vi "Calibrate_Test_Sums.vi"(8 "error in (no error)":errorcluster, 11 "StageSelection":enum16{"X-Y", "Z"}(ring)) -> (0 "error out":errorcluster)   [LabVIEW 2020]
doc: "Use this template to create a dialog box with event handling."
uses:
  Globals/gl_Calibration globals.vi
  Typedefs/Top level VI states.ctl
panel:
  out "Znorm_to_um_scaling":dbl
  in  "Delay":u32=1000
  out "Cal":sgl[][](array[numeric])
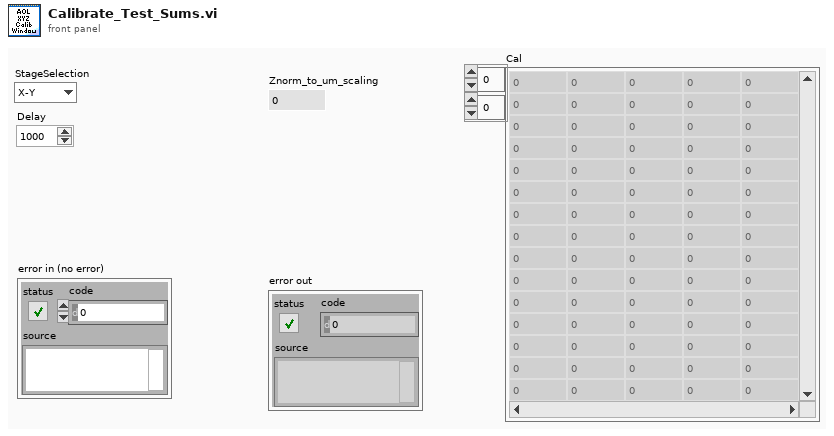
[diagram p1: front panel]
types:
  T1 = typedef "Cal points.ctl" = enum16{"5-points calibration (crude)", "11-points calibration", "21-points calibration", "41-points calibration"}
  T2 = typedef "Top level VI states.ctl" = enum16{"None", "Initialise UI", "<STACK PROTOCOL STATES>", "AOL Zstack-START", "AOL Zstack-STOP", "Motor Zstack-START", "Motor Zstack-STOP", "<ACQUISITION PROTOCOL STATES> ", "Functional Acquisition-START", "Functional Acquisition-STOP", "Single Plane Acquisition-START", "Single Plane Acquisition-STOP", "Volume Acquisition-START", "Volume Acquisition-STOP", "<LIVE IMAGING PROTOCOL STATES>", "Live Imaging-START", "Live Imaging-STOP", "Live Plane Imaging-START", "Live Plane Imaging-STOP", "Live Volume Imaging-START", "Live Volume Imaging-STOP", "<MOVEMENT CORRECTION PROTOCOL STATES>", "EXIT"}
  T3 = typedef "General Scan Parameters.ctl" = cluster{"Field of View":sgl, "Frame Size":u16, "Dwell Time (ms)":dbl, "Wavelength (nm)":dbl, "Zoom":dbl, "AOL Xc":sgl, "AOL Yc":sgl, "AOL Zc":sgl, "AOL Mode":enum16{"Raster", "Structural", "Pointing", "Mini Scan", "Alignment"}, "Imaging Mode":enum16{"Live Imaging", "AOL Zstack", "Motor Zstack", "Functional Imaging"}}
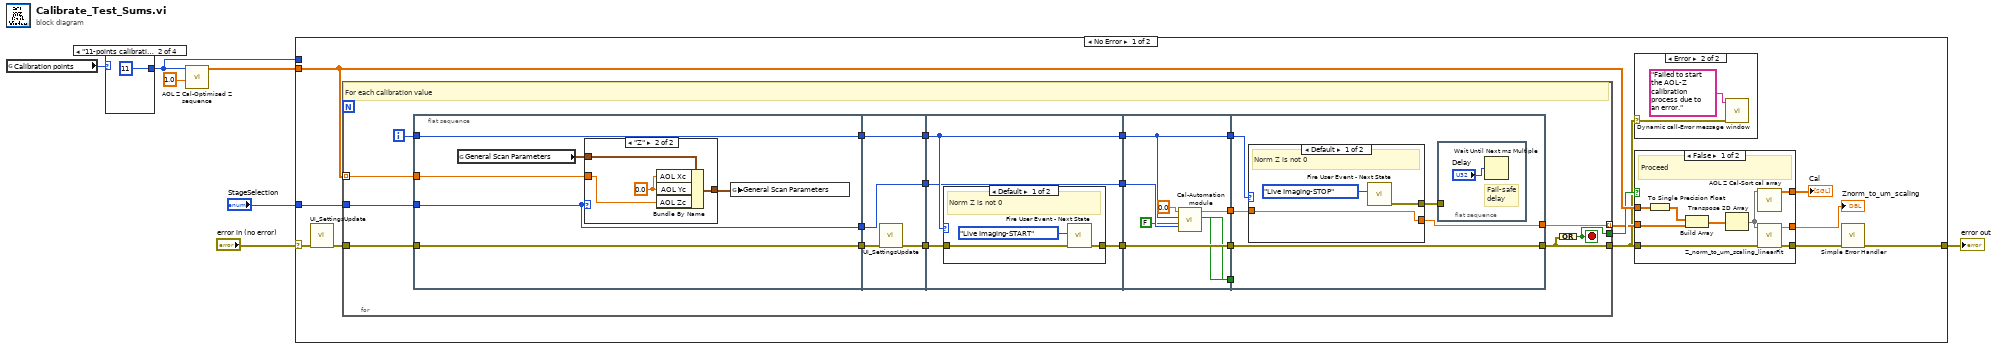
[diagram p0: block diagram]
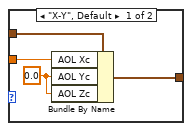
[diagram p2: hidden frame]
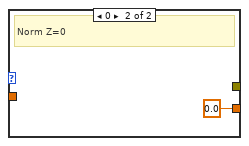
[diagram p4: hidden frame]
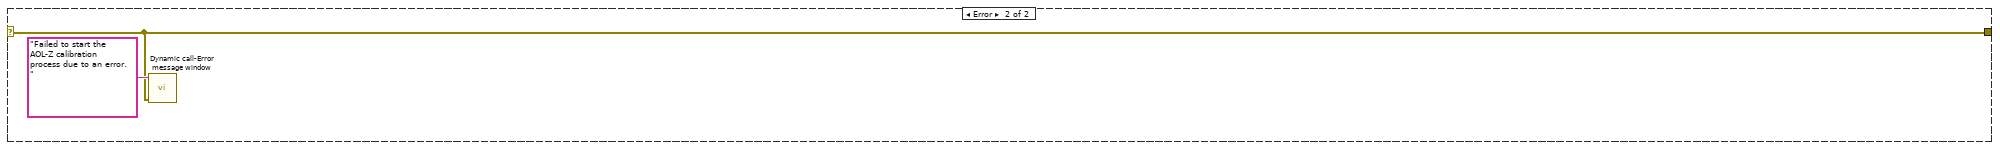
[diagram p7: hidden frame]
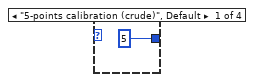
[diagram p8: hidden frame]
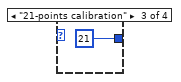
[diagram p9: hidden frame]
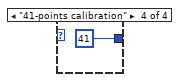
[diagram p10: hidden frame]
diagram:
  n1 = global read "gl_Calibration globals.vi" "Calibration points"() -> (w5:T1)
  n2 = case shown="\"11-points calibration\"" w5 {
    tunnel: [5 ("Calibration points") 11 ("Calibration points") 21 ("Calibration points") 41 ("Calibration points")] -> w4
    frame "5-points calibration (crude)", Default {
    }
    frame "11-points calibration" {
    }
    frame "21-points calibration" {
    }
    frame "41-points calibration" {
    }
  }
  n3 = call "AOL Z Cal-Optimised Z sequence.vi"("Max positive value"=1.0, "Calibration points"=w4) -> ("Calibration's optimised norm Z sequence"=w7:dbl[])  [unwired: 8 in, 1 out]
  n4 = case shown="No Error" "error in (no error)" {
    selector: "error in (no error)" -> [w15 w100]
    tunnel: w7 -> [w22 _]
    tunnel: w4 -> [_ _]
    tunnel: [w18 w100] -> w3
    tunnel: "StageSelection" -> [w13 _]
    frame No Error {
      n5 = call "UI_SettingsUpdate.vi"("error in (no error)"=w15) -> ("error out"=w17:errorcluster)  [unwired: 10 in]
      n6 = for {
        tunnel: w22 -> [w38] mode=indexing
        tunnel: [w43] -> w16 mode=indexing
        tunnel: [w25] -> w19
        tunnel: [w26] -> w14
        tunnel: w17 -> [w34]
        tunnel: w13 -> [w32]
        i -> [w35]
        stop <- w25 stop-if-true
        # "For each calibration value"
        n7 = flat-sequence {
          tunnel: w35 -> [w49]
          tunnel: [w49] -> w39
          tunnel: w38 -> [w45]
          tunnel: w34 -> [w48]
          tunnel: [w48] -> w33
          tunnel: w32 -> [w44]
          tunnel: [w44] -> w28
          tunnel: [w61] -> w41
          tunnel: w39 -> [w61]
          tunnel: w33 -> [w60]
          tunnel: [w59] -> w31
          tunnel: [w58] -> w29
          tunnel: w28 -> [w58]
          tunnel: [w65] -> w42
          tunnel: w41 -> [w65]
          tunnel: [w64] -> w36
          tunnel: w31 -> [w63]
          tunnel: [w62] -> w30
          tunnel: w29 -> [w62]
          tunnel: w42 -> [w74]
          tunnel: [w76] -> w40
          tunnel: [w77] -> w37
          tunnel: w36 -> [w77]
          tunnel: w30 -> [w75]
          tunnel: [w74] -> w27
          tunnel: [w71] -> w24
          tunnel: [w70] -> w23
          tunnel: [w81] -> w43
          tunnel: w40 -> [w80]
          tunnel: w37 -> [w79]
          tunnel: [w79] -> w26
          tunnel: w27 -> [w78]
          tunnel: w24 -> [_]
          tunnel: w23 -> [_]
          frame #0 {
            n8 = global read "gl_Calibration globals.vi" "General Scan Parameters"() -> (w47:T3)
            n9 = case shown="\"Z\"" w44 {
              tunnel: w47 -> [w50 w57]
              tunnel: [w53 w56] -> w46
              tunnel: w45 -> [w52 w54]
              frame "X-Y", Default {
                w51 = sgl 0.0 ("AOL Yc")
                n10 = Bundle By Name(cluster=w50, "AOL Xc"=w52, "AOL Yc"=w51, "AOL Zc"=w51) -> (w53:T3)
              }
              frame "Z" {
                w55 = sgl 0.0 ("AOL Xc")
                n11 = Bundle By Name(cluster=w57, "AOL Xc"=w55, "AOL Yc"=w55, "AOL Zc"=w54) -> (w56:T3)
              }
            }
            n12 = global write "gl_Calibration globals.vi" "General Scan Parameters"(w46) -> ()
          }
          frame #1 {
            n13 = call "UI_SettingsUpdate.vi"("error in (no error)"=w60) -> ("error out"=w59:errorcluster)  [unwired: 10 in]
          }
          frame #2 {
            n14 = case shown="Default" w65 {
              tunnel: [w67 w69] -> w64
              tunnel: w63 -> [w66 w69]
              frame Default {
                # "Norm Z is not 0"
                n15 = call "Fire User Event - Next State.vi"("Error In"=w66, "\"UI Handler loop\" case to execute"=Top_level_VI_states."Live Imaging-START" ("\"UI Handler loop\" case to execute")) -> ("Error Out"=w67:errorcluster)  [unwired: 9 in]
              }
              frame 0 {
                # "Norm Z=0"
              }
            }
          }
          frame #3 {
            n16 = call "Cal-Automation module.vi"(6:w75, "Timed out while waiting for acknowledgement in"=FALSE, "FOR loop index"=w74, "Initial motor position (um)"=sgl 0.0) -> ("Motor timed out or errored out"=w71:bool, "Cancelled"=w70:bool, "Measured cal value"=w76:sgl)  [unwired: 4 in, 1 out]
          }
          frame #4 {
            n17 = case shown="Default" w78 {
              tunnel: [w85 _] -> w82
              tunnel: [w84 sgl 0.0 ("Z")] -> w81
              tunnel: w80 -> [w84 _]
              frame Default {
                # "Norm Z is not 0"
                n18 = call "Fire User Event - Next State.vi"("\"UI Handler loop\" case to execute"=Top_level_VI_states."Live Imaging-STOP" ("\"UI Handler loop\" case to execute")) -> ("Error Out"=w85:errorcluster)  [unwired: 10 in]
              }
              frame 0 {
                # "Norm Z=0"
              }
            }
            n19 = flat-sequence {
              tunnel: w82 -> [_]
              frame #0 {
                # "Fail-safe delay"
                n20 = Wait Until Next ms Multiple(millisecond multiple="Delay") -> ()  [unwired: 1 out]
              }
            }
          }
        }
        n21 = Compound Arithmetic op=OR(w26) -> (w25:bool)
      }
      n22 = case shown="Error" w14 {
        selector: w14 -> [_ w89]
        frame No Error {
        }
        frame Error {
          n23 = call "Dynamic call-Error message window.vi"("error in (no error)"=w89, "Error Message"="Failed to start the AOL-Z calibration process due to an error.") -> ()  [unwired: 9 in, 1 out]
        }
      }
      n24 = case shown="False" w19 {
        tunnel: w22 -> [w98 _]
        tunnel: w16 -> [w97 _]
        tunnel: [w95 _] -> w21
        tunnel: [w93 w99] -> w20
        tunnel: w14 -> [w92 w99]
        tunnel: [w90 _] -> w12
        frame False {
          # "Proceed"
          n25 = To Single Precision Float(number=w98) -> (single precision float=w94:sgl[])
          n26 = Build Array(w94, w97) -> (w96:sgl[][])
          n27 = Transpose 2D Array(2D array=w96) -> (transposed array=w91:sgl[][])
          n28 = call "AOL Z Cal-Sort cal array.vi"("Unsorted cal"=w91) -> ("Sorted cal"=w95:sgl[][])  [unwired: 10 in]
          n29 = call "Z_norm_to_um_scaling_linearFit.vi"("Input Array(Znorm, Z_um)"=w91, "error in (no error)"=w92) -> ("Znorm_to_um_scaling"=w90:dbl, "error out"=w93:errorcluster)  [unwired: 7 in]
        }
        frame True {
          # "Cancelled/Aborted"
        }
      }
      "Cal" <- w21
      "Znorm_to_um_scaling" <- w12
      n30 = call <vilib>:"Simple Error Handler.vi"("error in (no error)"=w20) -> ("error out"=w18:errorcluster)  [unwired: 4 in, 4 out]
    }
    frame Error {
      n31 = call "Dynamic call-Error message window.vi"("error in (no error)"=w100, "Error Message"="Failed to start the AOL-Z calibration process due to an error.") -> ()  [unwired: 9 in, 1 out]
    }
  }
  "error out" <- w3
